vi "read binary advanced.vi"() -> ()   [LabVIEW 2016]
panel:
  out "Waveform Graph":dbl[](graph)
  out "Array from file":dbl[](array[numeric])
  in  "Read to Data point #":i32
  in  "Read from Data point #":i32
  in  "Read all points?":bool=TRUE
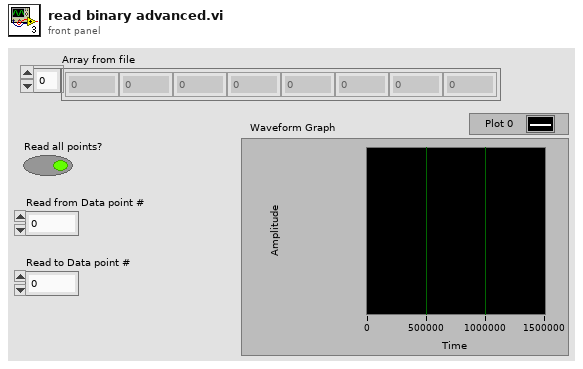
[diagram p1: front panel]
types:
  T1 = enum16{"big-endian, network order", "native, host order", "little-endian"}
  T2 = enum16{"deny read/write", "deny write-only", "deny none"}
  T3 = enum16{"open", "replace", "create", "open or create", "replace or create", "replace or create with confirmation"}
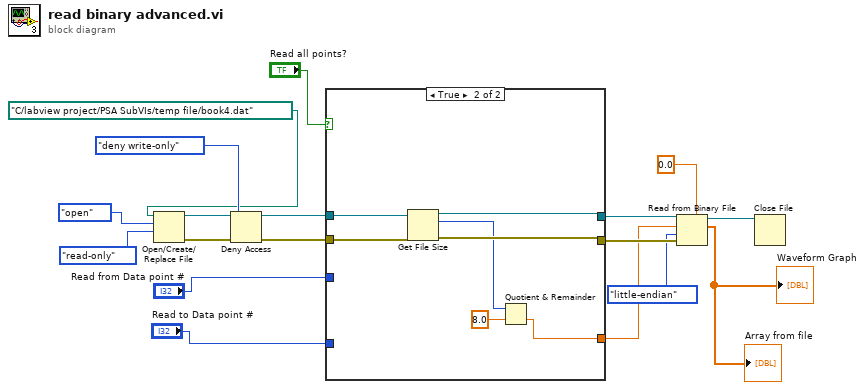
[diagram p0: block diagram]
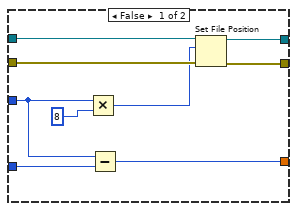
[diagram p2: hidden frame]
diagram:
  n1 = Open/Create/Replace File(file path (use dialog)=path "C:/labview project/PSA SubVIs/temp file/book4.dat", operation (0:open)=T3."open", access (0:read/write)=enum16{"read/write", "read-only", "write-only"}."read-only") -> (refnum out=w15:refnum<file>, error out=w14:errorcluster)  [unwired: 3 in, 1 out]
  n2 = Deny Access(4:w14, 6:T2."deny write-only" ("deny mode (0:deny read/write)"), 7:w15) -> (0:w11:errorcluster, 3:w12:refnum<file>)
  n3 = case shown="True" "Read all points?" {
    tunnel: w12 -> [w27 w34]
    tunnel: w11 -> [w26 w33]
    tunnel: "Read from Data point #" -> [w21 _]
    tunnel: [w23 w32] -> w9
    tunnel: [w22 w31] -> w8
    tunnel: "Read to Data point #" -> [w20 _]
    tunnel: [w19 w29] -> w6
    frame False {
      n4 = Multiply(x=w21, y=8) -> (x*y=w24:i32)
      n5 = Subtract(x=w21, y=w20) -> (x-y=w19:i32)
      n6 = Set File Position(offset (in bytes) (0)=w24, refnum=w27, error in=w26) -> (refnum out=w23:refnum<file>, error out=w22:errorcluster)  [unwired: 1 in]
    }
    frame True {
      n7 = Get File Size(file=w34, error in=w33) -> (refnum out=w32:refnum<file>, size (in bytes)=w28:i64, 0:w31:errorcluster)
      n8 = Quotient & Remainder(x=w28, y=8.0) -> (floor(x/y)=w29:dbl)  [unwired: 1 out]
    }
  }
  n9 = Read from Binary File(5:0.0, 8:w8, 9:T1."little-endian" ("byte order (0:big-endian, network order)"), 10:w6, 11:w9) -> (2:→"Array from file" →"Waveform Graph":dbl[], 3:w4:refnum<file>)  [unwired: 1 in, 2 out]
  n10 = Close File(refnum=w4) -> ()  [unwired: 1 in, 2 out]
